vi "DataFile _ Read INI File.vi"(8 "error in":errorcluster, 11 "configuration file path":path) -> (0 "error out":errorcluster, 2 "value":T1)   [LabVIEW 2016]
uses:
  <vilib>/Utility/config.llb/Read Key (Path).vi
  <vilib>/Utility/config.llb/Read Key (String).vi
  <vilib>/Utility/config.llb/Read Key (I32).vi
  <vilib>/Utility/config.llb/NI_LVConfig.lvlib
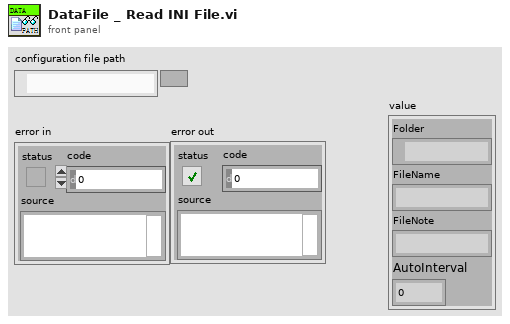
[diagram p1: front panel]
types:
  T1 = cluster{"Folder":path, "FileName":string, "FileNote":string, "AutoInterval":i32}
  T2 = typedef "NI_LVConfig.lvlib/Config Data RefNum.ctl" = refnum<k1>
  T3 = cluster{"value":path, "value":string, "value":string, "value":i32}
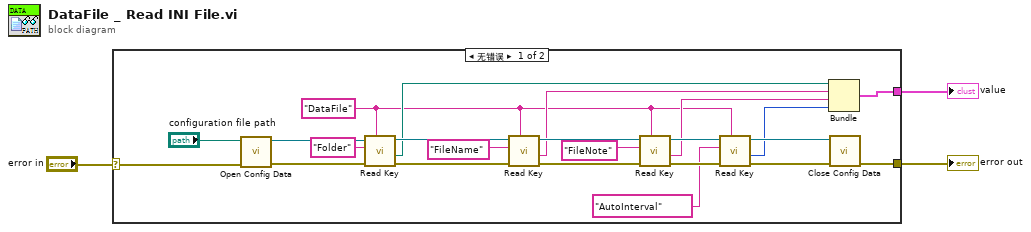
[diagram p0: block diagram]
diagram:
  n1 = case shown="无错误" "error in" {
    selector: "error in" -> [w18 w27]
    tunnel: [w17 w27] -> w2
    tunnel: [w14 _] -> w1
    frame No Error {
      w6 = "DataFile" ("section")
      n2 = call <vilib>:"Open Config Data.vi"("error in (no error)"=w18, "configuration file path"="configuration file path") -> ("error out"=w25:errorcluster, "refnum"=w26:T2)  [unwired: 7 in, 1 out]
      n3 = call-poly <vilib>:"Read Key.vi"("section"=w6, "error in (no error)"=w25, "key"="Folder", "refnum"=w26) -> ("error out"=w23:errorcluster, "value"=w16:path, "refnum out"=w22:T2)  [unwired: 4 in, 1 out]
      n4 = call-poly <vilib>:"Read Key.vi"("section"=w6, "error in (no error)"=w23, "key"="FileName", "refnum"=w22) -> ("error out"=w12:errorcluster, "value"=w15:string, "refnum out"=w20:T2)  [unwired: 4 in, 1 out]
      n5 = call-poly <vilib>:"Read Key.vi"("section"=w6, "error in (no error)"=w12, "key"="FileNote", "refnum"=w20) -> ("error out"=w8:errorcluster, "value"=w10:string, "refnum out"=w13:T2)  [unwired: 4 in, 1 out]
      n6 = call-poly <vilib>:"Read Key.vi"("section"=w6, "error in (no error)"=w8, "key"="AutoInterval", "refnum"=w13) -> ("error out"=w7:errorcluster, "value"=w4:i32, "refnum out"=w9:T2)  [unwired: 4 in, 1 out]
      n7 = Bundle("value"=w16, "value"=w15, "value"=w10, "value"=w4) -> (w14:T3)  [unwired: 1 in]
      n8 = call <vilib>:"Close Config Data.vi"("error in (no error)"=w7, "refnum"=w9) -> ("error out"=w17:errorcluster)  [unwired: 8 in, 1 out]
    }
    frame Error {
    }
  }
  "error out" <- w2
  "value" <- w1
